vi "Remove NaNs.vi"(3 "Sinusoid":dbl[][](array[numeric]) format="%.2f", 4 "Response":dbl[](array[numeric]) format="%.2f", 5 "Stimulus":dbl[](array[numeric]) format="%.2f") -> (0 "Sinusoid (out)":dbl[][](array[numeric]) format="%.2f", 1 "Response (out)":dbl[](array[numeric]) format="%.2f", 2 "Stimulus (out)":dbl[](array[numeric]) format="%.2f")   [LabVIEW 2013, in "nan operations.lvlib"]
uses:
  nan operations.lvlib
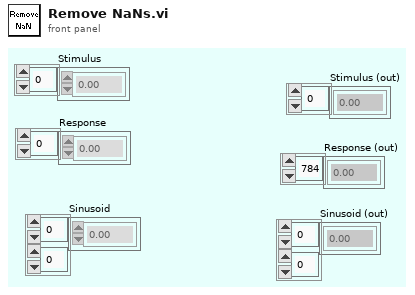
[diagram p1: front panel]
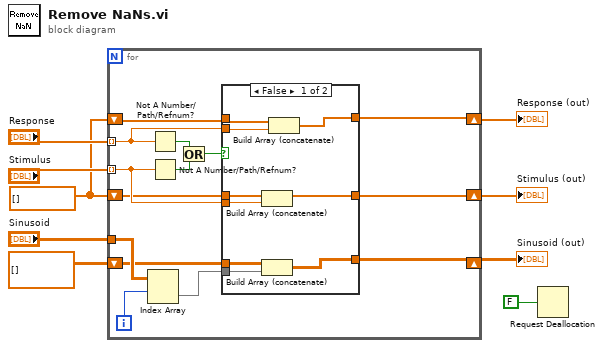
[diagram p0: block diagram]
diagram:
  w5 = dbl[] [] ("subarray")
  n1 = for {
    tunnel: "Response" -> [w23] mode=indexing
    tunnel: "Stimulus" -> [w18] mode=indexing
    shift-right: [w12] -> w4
    shift-left: w5 -> [w19]
    shift-right: [w16] -> w2
    shift-left: w5 -> [w17]
    shift-right: [w13] -> w3
    shift-left: dbl[][] [] ("subarray") -> [w14]
    tunnel: "Sinusoid" -> [w15]
    i -> [w10]
    n2 = Index Array(array=w15, index (row)=w10) -> (element=w11:dbl[])  [unwired: 1 in]
    n3 = Not A Number/Path/Refnum?(number/path/refnum=w23) -> (NaN/Path/Refnum?=w21:bool)
    n4 = Not A Number/Path/Refnum?(number/path/refnum=w18) -> (NaN/Path/Refnum?=w22:bool)
    n5 = Or(x=w21, y=w22) -> (x .or. y?=w20:bool)
    n6 = case shown="False" w20 {
      tunnel: w19 -> [w27 w35]
      tunnel: [w32 w35] -> w12
      tunnel: w23 -> [w26 _]
      tunnel: w18 -> [w25 _]
      tunnel: w17 -> [w31 w34]
      tunnel: [w30 w34] -> w16
      tunnel: w11 -> [w24 _]
      tunnel: w14 -> [w29 w33]
      tunnel: [w28 w33] -> w13
      frame False {
        n7 = Build Array (concatenate)(w31, w25) -> (w30:dbl[])
        n8 = Build Array (concatenate)(w29, w24) -> (w28:dbl[][])
        n9 = Build Array (concatenate)(w27, w26) -> (w32:dbl[])
      }
      frame True {
      }
    }
  }
  "Response (out)" <- w4
  "Sinusoid (out)" <- w3
  "Stimulus (out)" <- w2
  n10 = Request Deallocation(FALSE ("flag")) -> ()
